vi "Siargo Stop.vi"(8 "error in":errorcluster, 11 "Modbus master in":refnum<class "Modbus Master.lvclass">) -> (0 "error out":errorcluster)   [LabVIEW 2020]
uses:
  <vilib>/NI/Modbus Library/API/Master/Modbus Master.lvclass
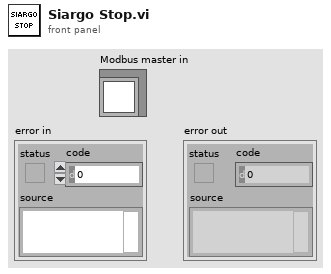
[diagram p1: front panel]
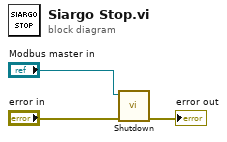
[diagram p0: block diagram]
diagram:
  n1 = call-dynamic "Shutdown.vi"("error in"="error in", "Modbus master in"="Modbus master in") -> ("error out"=→"error out":errorcluster)  [unwired: 9 in]
